vi "dscOutp.vi"(8 "error in":errorcluster, 10 "valueIn":u8, 11 "addressIn":u32) -> (0 "error out":errorcluster, 2 "value":u8, 3 "addressOut":u32)   [LabVIEW 2011, in "Diamond Universal Driver.lvlib"]
doc: "Board independent direct I/O. Write a byte to that address."
uses:
  Diamond Universal Driver.lvlib
  Instruments/WL OPC/Support/dlls/dscud.dll
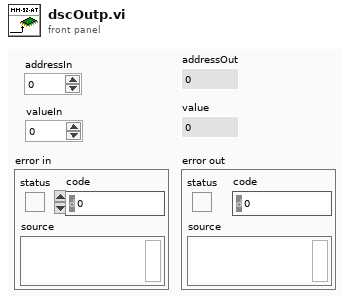
[diagram p1: front panel]
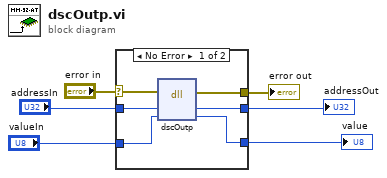
[diagram p0: block diagram]
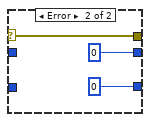
[diagram p2: hidden frame]
diagram:
  n1 = case shown="No Error" "error in" {
    selector: "error in" -> [w12 w15]
    tunnel: [w8 w15] -> w5
    tunnel: [w11 u32 0 ("address")] -> w4
    tunnel: [w10 u8 0 ("value")] -> w3
    tunnel: "addressIn" -> [w9 _]
    tunnel: "valueIn" -> [w7 _]
    frame No Error {
      n2 = dll-call lib="C:/Users/mrichardson/Documents/Web Based Version Control SW/Instruments/WL OPC/Support/dlls/dscud.dll" fn="dscOutp"(error in=w12, "address"=w9, "value"=w7) -> (error out=w8:errorcluster, "address"=w11:u32, "value"=w10:u8)  [unwired: 3 in, 1 out]
    }
    frame Error {
    }
  }
  "value" <- w3
  "addressOut" <- w4
  "error out" <- w5
